vi "Mapeo LabView.vi"() -> ()   [LabVIEW 2013]
panel:
  in  "stop":bool
  out "output variable":dbl
  in  "Slide":dbl(slide) scale=0.0..583.0
  # "D"
  # "A"
  # "E"
  # "B"
  # "C"
  # "long map(long x, long in_min, long in_max, long out_min, long out_max)\n{\n  return (x - in_min) * (out_max - out_min) / (in_max - in_min) + out_min;\n}"
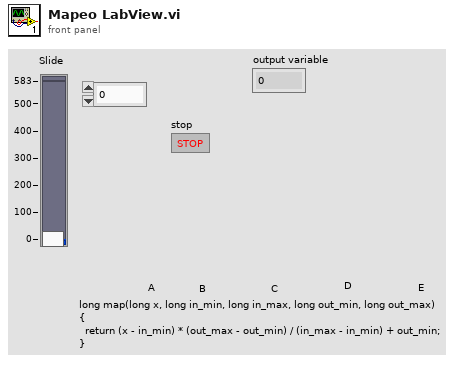
[diagram p1: front panel]
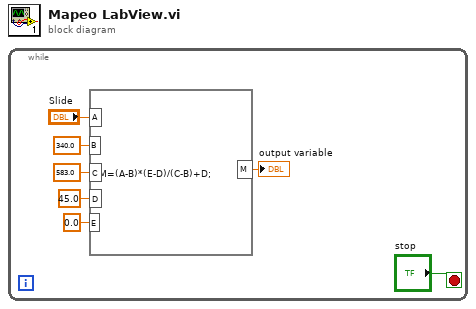
[diagram p0: block diagram]
diagram:
  n1 = while {
    stop <- "stop" stop-if-true
    n2 = formula code="M=(A-B)*(E-D)/(C-B)+D;"("A"="Slide", "B"=340.0 ("input variable"), "C"=583.0 ("input variable"), "D"=45.0 ("input variable"), "E"=0.0 ("input variable")) -> ("M"=→"output variable":dbl)
  }
